vi "SS_DeleteLocalFile.vi"(6 "Main Cluster IN":T1, 8 "Error In":errorcluster, 11 "Info In":string="\nWaiting for TimerScope Trigger\n- IN: SS TimerScope Trigger\n- OUT: SET SS ThermoRec Received Trigger\nPulse Number is 231123\nPulse Type is 4\n\nDuration (s) is  2.000000\nDelay (s)  is  1.000000\nScan Period (ms) is  15\nNumber of Samples is  134\n\nDelay Started\nDelay Complete\nExternal Measurement of Delay (s): 1.000000\nACQUIRING DATA") -> (0 "Error Out":errorcluster, 3 "Info Out":string="\nWaiting for TimerScope Trigger\n- IN: SS TimerScope Trigger\n- OUT: SET SS ThermoRec Received Trigger\nPulse Number is 231123\nPulse Type is 4\n\nDuration (s) is  2.000000\nDelay (s)  is  1.000000\nScan Period (ms) is  15\nNumber of Samples is  134\n\nDelay Started\nDelay Complete\nExternal Measurement of Delay (s): 1.000000\nACQUIRING DATA", 4 "Main Cluster OUT":T1)   [LabVIEW 2016]
uses:
  Control/Control_Main.ctl
  Control/Control_ModuleArray.ctl
panel:
  in  "Tab Control":enum32{"IN", "OUT", "SubVI Info"}(tab)
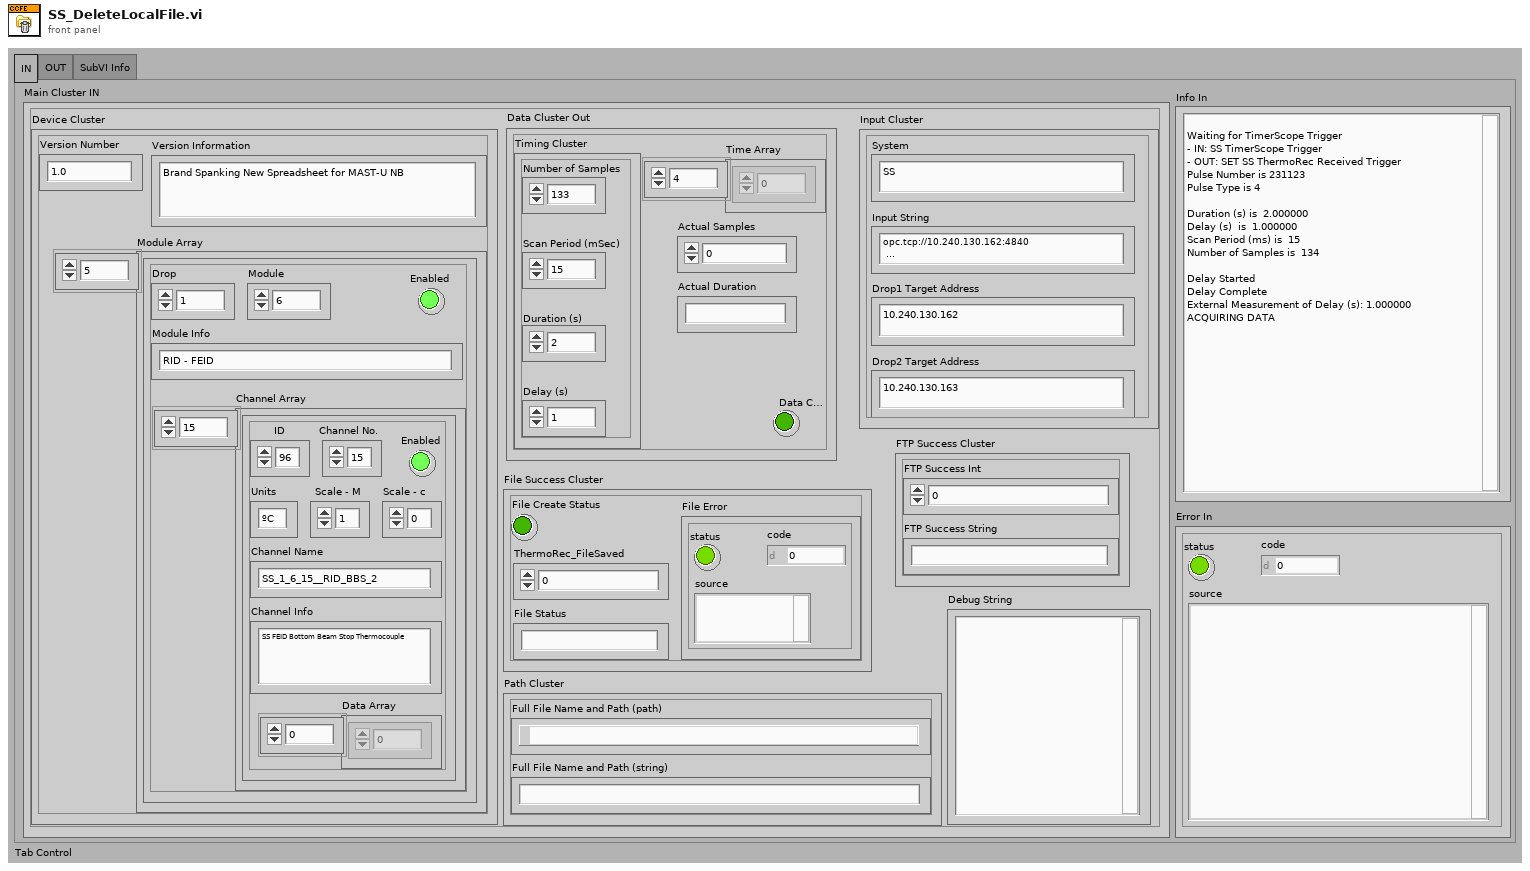
[diagram p1: front panel]
types:
  T1 = typedef "Control_Main.ctl" = cluster{"Device Cluster":cluster{"Module Array":T2, "Version Number":string, "Version Information":string}, "Input Cluster":cluster{"Input String":string, "Drop1 Target Address":string, "Drop2 Target Address":string, "System":string}, "Data Cluster Out":cluster{"Timing Cluster":cluster{"Number of Samples":i32, "Scan Period (mSec)":u32, "Duration (s)":dbl, "Delay (s)":dbl}, "Time Array":dbl[], "Actual Samples":i32, "Actual Duration":string, "Data Collection Error":bool}, "Path Cluster":cluster{"Full File Name and Path (path)":path, "Full File Name and Path (string)":string}, "File Success Cluster":cluster{"ThermoRec_FileSaved":i32, "File Create Status":bool, "File Error":errorcluster, "File Status":string}, "FTP Success Cluster":cluster{"FTP Success Int":i32, "FTP Success String":string}, "Debug String":string}
  T2 = typedef "Control_ModuleArray.ctl" = cluster{"Drop":i32, "Module":i32, "Module Info":string, "Enabled":bool, "Channel Array":cluster{"ID":i32, "Channel No.":i32, "Enabled":bool, "Channel Name":string, "Channel Info":string, "Units":string, "Scale - M":dbl, "Scale - c":dbl, "Data Array":dbl[]}[]}[]
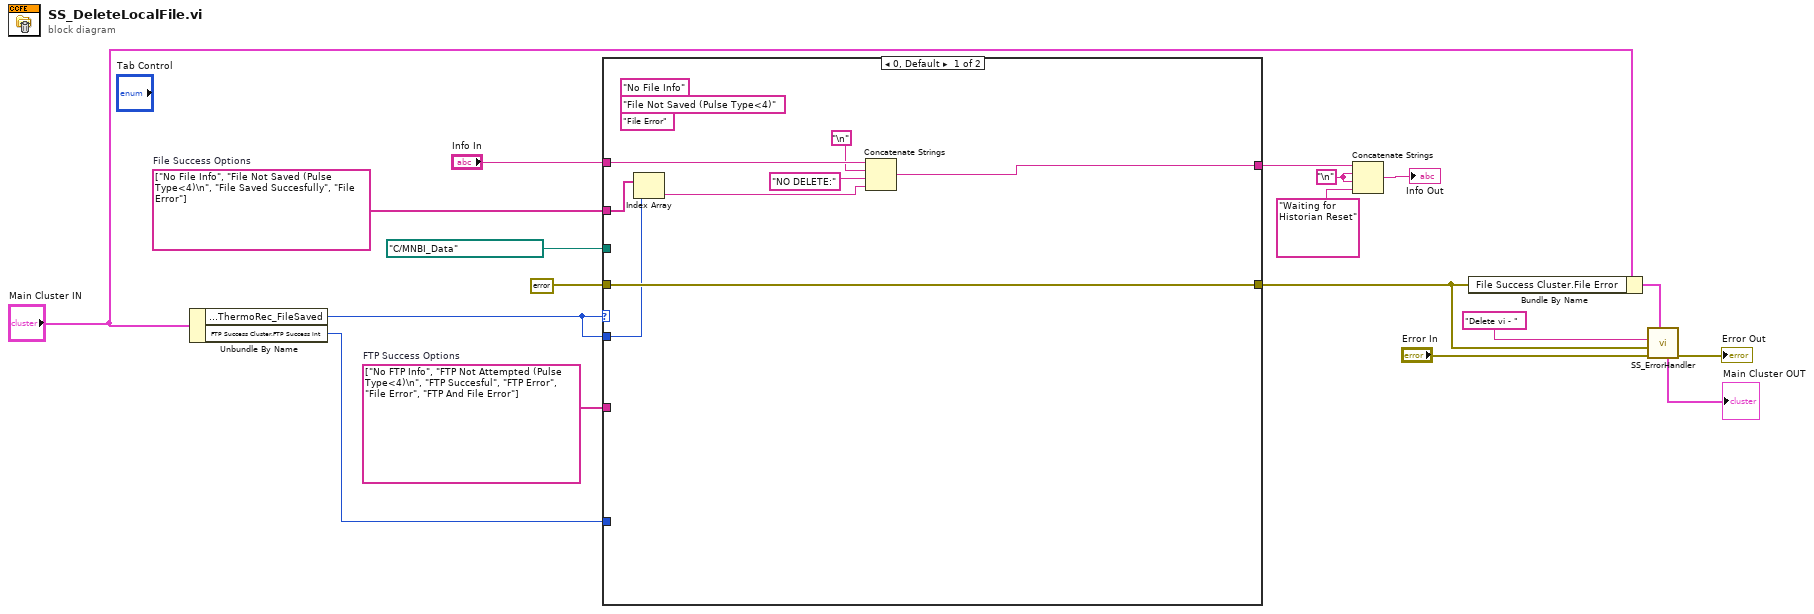
[diagram p0: block diagram]
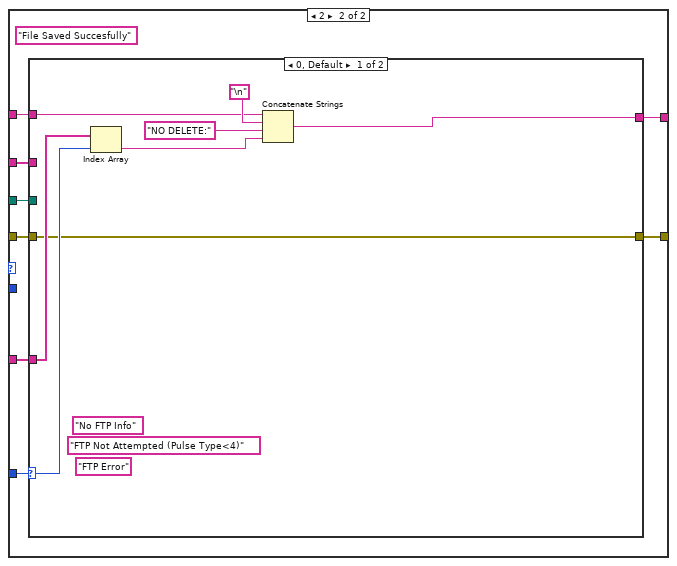
[diagram p2: hidden frame]
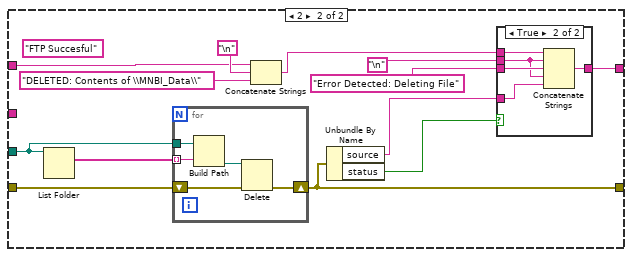
[diagram p3: hidden frame]
diagram:
  w14 = "\n"
  w17 = string[] ["No File Info", "File Not Saved (Pulse Type<4)\n", "File Saved Succesfully", "File Error"]  # File Success Options
  w16 = string[] ["No FTP Info", "FTP Not Attempted (Pulse Type<4)\n", "FTP Succesful", "FTP Error", "File Error", "FTP And File Error"]  # FTP Success Options
  n1 = Unbundle By Name("Main Cluster IN") -> ("File Success Cluster.ThermoRec_FileSaved"=w11:i32, "FTP Success Cluster.FTP Success Int"=w10:i32)
  n2 = case shown="0, Default" w11 {
    tunnel: "Info In" -> [w25 w31]
    tunnel: [w24 w30] -> w12
    tunnel: path "C:/MNBI_Data" ("path") -> [_ w29]
    tunnel: w10 -> [_ w34]
    tunnel: w17 -> [w26 w33]
    tunnel: w16 -> [_ w32]
    tunnel: [w20 w28] -> w3
    tunnel: errorcluster {"status"=FALSE, "code"=0, "source"=""} ("Error Out 2") -> [w20 w27]
    tunnel: w11 -> [w19 _]
    frame 0, Default {
      (unwired) "File Error"
      (unwired) "File Not Saved (Pulse Type<4)"
      (unwired) "No File Info"
      n3 = Index Array(array=w26, index=w19) -> (element=w21:string)
      n4 = Concatenate Strings(w25, "\n", "NO DELETE:", w21) -> (w24:string)
    }
    frame 2 {
      (unwired) "File Saved Succesfully"
      n5 = case shown="0, Default" w34 {
        selector: w34 -> [w37 _]
        tunnel: w33 -> [_ _]
        tunnel: w32 -> [w38 _]
        tunnel: w31 -> [w39 w53]
        tunnel: [w36 w43] -> w30
        tunnel: w29 -> [_ w51]
        tunnel: [w35 w49] -> w28
        tunnel: w27 -> [w35 w50]
        frame 0, Default {
          (unwired) "FTP Error"
          (unwired) "FTP Not Attempted (Pulse Type<4)"
          (unwired) "No FTP Info"
          n6 = Index Array(array=w38, index=w37) -> (element=w40:string)
          n7 = Concatenate Strings(w39, "\n", "NO DELETE:", w40) -> (w36:string)
        }
        frame 2 {
          (unwired) "FTP Succesful"
          n8 = List Folder(path=w51) -> (filenames=w52:string[])  [unwired: 3 in, 3 out]
          n9 = for {
            tunnel: w52 -> [w65] mode=indexing
            tunnel: w51 -> [w66]
            shift-right: [w63] -> w49
            shift-left: w50 -> [w62]
            n10 = Build Path(base path=w66, name or relative path=w65) -> (appended path=w64:path)
            n11 = Delete(path (use dialog)=w64, error in=w62) -> (error out=w63:errorcluster)  [unwired: 3 in, 2 out]
          }
          n12 = Concatenate Strings(w53, "\n", "DELETED: Contents of \\MNBI_Data\\") -> (w46:string)
          n13 = Unbundle By Name(w49) -> ("source"=w47:string, "status"=w48:bool)
          n14 = case shown="True" w48 {
            tunnel: [w56 w61] -> w43
            tunnel: w47 -> [_ w57]
            tunnel: w46 -> [w56 w60]
            tunnel: "\n" -> [_ w58]
            tunnel: "Error Detected: Deleting File" -> [_ w59]
            frame False {
            }
            frame True {
              n15 = Concatenate Strings(w60, w58, w59, w58, w57) -> (w61:string)
            }
          }
        }
      }
    }
  }
  n16 = Concatenate Strings(w12, w14, w14, "Waiting for Historian Reset") -> (→"Info Out":string)
  n17 = Bundle By Name(cluster="Main Cluster IN", "File Success Cluster.File Error"=w3) -> (w2:T1)
  n18 = call "SS_ErrorHandler.vi"("Main Cluster IN"=w2, "Error In"="Error In", "SubVI Error"=w3, "SubVI Name"="Delete vi - ") -> ("Error Out"=→"Error Out":errorcluster, "Main Cluster OUT"=→"Main Cluster OUT":T1)  [unwired: 5 in, 1 out]
